vi "VFH.vi"(8 "Previous Calculated Sector":i16=90, 9 "Compass Bearing (degrees)":dbl, 10 "Target Bearing (degrees)":dbl, 11 "RAW SICK Data":T1) -> (3 "Calculated sector":i16)   [LabVIEW 2009]
uses:
  TypeDefs/Sensor TypeDefs/SICK Array.ctl
  Functional Global Variables/Actions for FG's.ctl
panel:
  in  "Roll offset":dbl
  in  "Pitch offset":dbl
  in  "Cost scaling factor":dbl=90.0
  in  "Heading scaling factor":dbl=5.0
  out "Number of Obstructed Sectors 3":i32
  out "Number of Obstructed Sectors 2":i32
  out "Number of Obstructed Sectors":i32
  out "Expansion Array 3":u16[](array[numeric])
  out "Expansion Array 2":u16[](array[numeric])
  out "Expansion Array":u16[](graph)
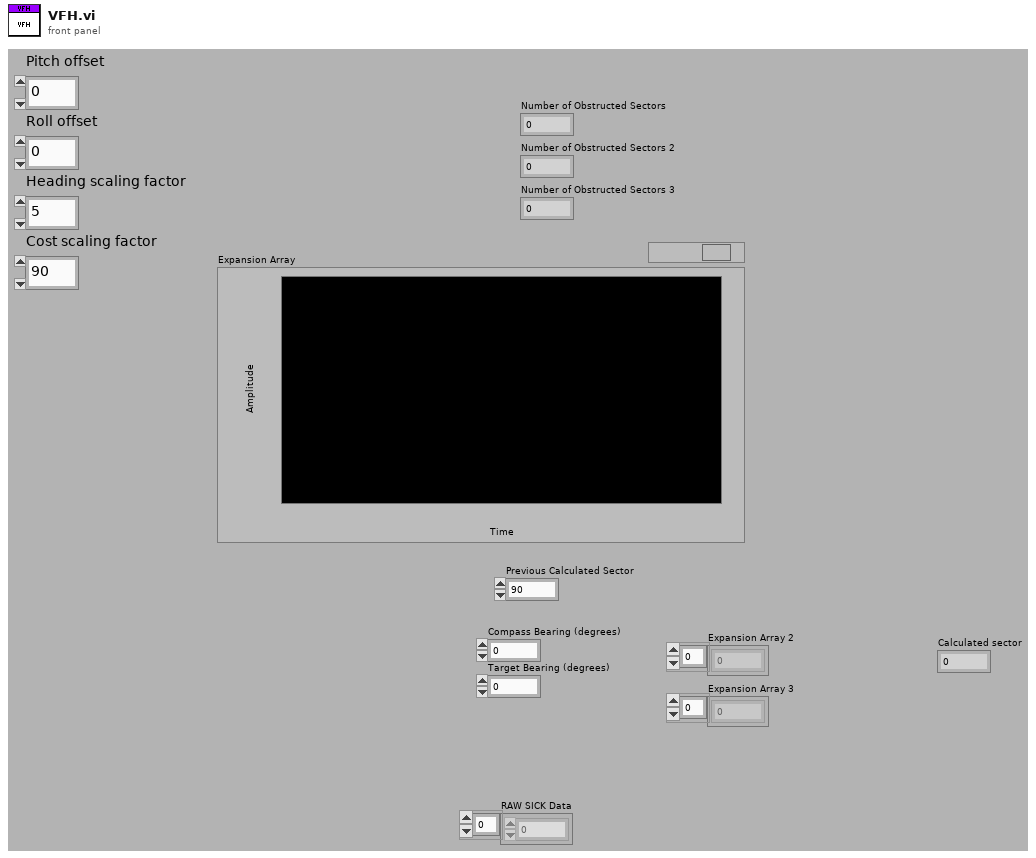
[diagram p1: front panel]
types:
  T1 = typedef "SICK Array.ctl" = u16[]
  T2 = typedef "Actions for FG's.ctl" = enum16{"Read", "Write"}
  T3 = typedef "VFH Parameters.ctl" = cluster{"Robot Radius":u16, "Near Threshold":u16, "Mid Threshold":u16, "Far Threshold":u16, "Weights":T4}
  T4 = typedef "VFH Weights.ctl" = cluster{"TS-S weight":dbl, "CS-S weight":dbl, "PCS-S weight":dbl, "Near weight":dbl, "Mid weight":dbl, "Far weight":dbl}
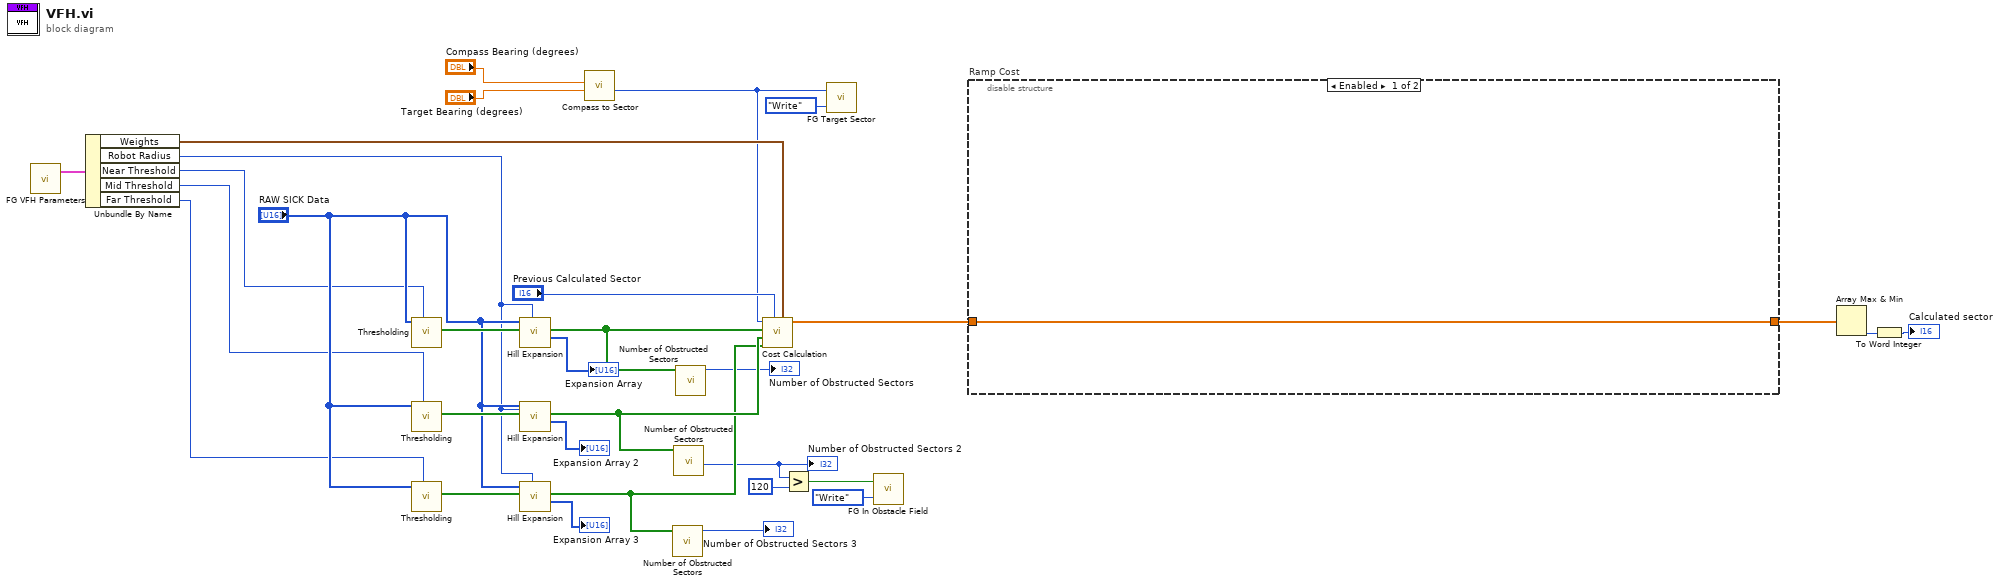
[diagram p0: block diagram]
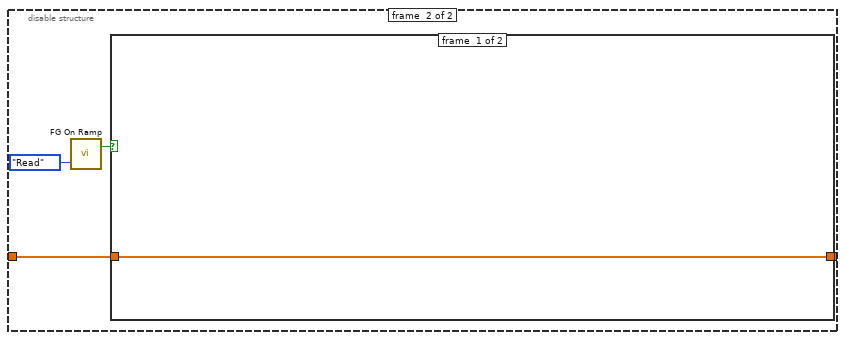
[diagram p2: hidden frame]
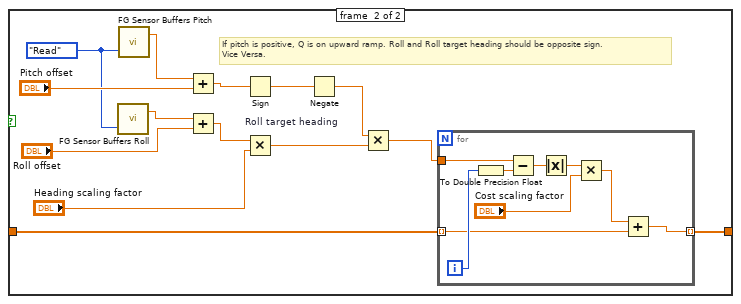
[diagram p3: hidden frame]
diagram:
  n1 = call "FG VFH Parameters.vi"() -> ("VFH Parameters out"=w23:T3)  [unwired: 3 in]
  n2 = Unbundle By Name(w23) -> ("Weights"=w18:T4, "Robot Radius"=w22:u16, "Near Threshold"=w21:u16, "Mid Threshold"=w20:u16, "Far Threshold"=w19:u16)
  n3 = call "Thresholding.vi"("Threshold"=w21, "RAW SICK Data"="RAW SICK Data") -> ("Boolean array"=w31:bool[])  [unwired: 1 in, 8 out]
  n4 = call "Thresholding.vi"("Threshold"=w20, "RAW SICK Data"="RAW SICK Data") -> ("Boolean array"=w29:bool[])  [unwired: 1 in, 8 out]
  n5 = call "Thresholding.vi"("Threshold"=w19, "RAW SICK Data"="RAW SICK Data") -> ("Boolean array"=w30:bool[])  [unwired: 1 in, 8 out]
  n6 = call "Hill Expansion.vi"("Robot Radius"=w22, "Boolean array"=w31, "RAW SICK Data"="RAW SICK Data") -> ("Expansion Array"=→"Expansion Array":u16[], "Expanded Boolean Array"=w11:bool[])  [unwired: 1 in, 6 out]
  n7 = call "Hill Expansion.vi"("Robot Radius"=w22, "Boolean array"=w29, "RAW SICK Data"="RAW SICK Data") -> ("Expansion Array"=→"Expansion Array 2":u16[], "Expanded Boolean Array"=w10:bool[])  [unwired: 1 in, 6 out]
  n8 = call "Hill Expansion.vi"("Robot Radius"=w22, "Boolean array"=w30, "RAW SICK Data"="RAW SICK Data") -> ("Expansion Array"=→"Expansion Array 3":u16[], "Expanded Boolean Array"=w9:bool[])  [unwired: 1 in, 6 out]
  n9 = call "Compass to Sector.vi"("Target Bearing (degrees)"="Target Bearing (degrees)", "Compass Bearing (degrees)"="Compass Bearing (degrees)") -> ("Target Heading (Sectors)"=w16:i16)  [unwired: 9 out]
  n10 = call "Number of Obstructed Sectors.vi"("Boolean Array"=w9) -> ("Number of Obstructed Sectors"=→"Number of Obstructed Sectors 3":i32)  [unwired: 10 in]
  n11 = call "Number of Obstructed Sectors.vi"("Boolean Array"=w10) -> ("Number of Obstructed Sectors"=w6:i32)  [unwired: 10 in]
  "Number of Obstructed Sectors 2" <- w6
  n12 = call "Number of Obstructed Sectors.vi"("Boolean Array"=w11) -> ("Number of Obstructed Sectors"=→"Number of Obstructed Sectors":i32)  [unwired: 10 in]
  n13 = call "Cost Calculation.vi"("Weights"=w18, "Previous Calculated Sector"="Previous Calculated Sector", "Far Boolean Array"=w9, "Mid Boolean Array"=w10, "Near Boolean Array"=w11, "Target Sector"=w16) -> ("Cost Array"=w2:dbl[])  [unwired: 5 in]
  n14 = Greater?(x=w6, y=120) -> (0:w4:bool)
  n15 = call "FG Target Sector.vi"("FG Action (Read)"=Actions_for_FG's."Write", "Target sector in"=w16) -> ()  [unwired: 1 in, 1 out]
  n16 = call "FG In Obstacle Field.vi"("FG Action (Read)"=Actions_for_FG's."Write", "In Obs. Field? in"=w4) -> ()  [unwired: 1 in, 1 out]
  n17 = disable-structure "Ramp Cost" shown="Enabled" {
    disable-tunnel: w2 -> [w32 w34]
    disable-tunnel: [w32 w33] -> w1
    frame #0 {
    }
    frame #1 {
      n18 = call "FG On Ramp.vi"("FG Action"=Actions_for_FG's."Read") -> ("On Ramp out"=w35:bool)  [unwired: 2 in]
      n19 = case shown="True" w35 {
        tunnel: w34 -> [w37 w50]
        tunnel: [w37 w49] -> w33
        frame #0 {
        }
        frame #1 {
          w42 = Actions_for_FG's."Read" ("FG Action (Read)")
          # "If pitch is positive, Q is on upward ramp. Roll and Roll target heading should be opposite sign.\nVice Versa."
          n20 = call "FG Sensor Buffers Roll.vi"("FG Action (Read)"=w42) -> ("Roll Buffer out"=w41:dbl)  [unwired: 2 in]
          n21 = call "FG Sensor Buffers Pitch.vi"("FG Action (Read)"=w42) -> ("Pitch Buffer out"=w44:dbl)  [unwired: 2 in]
          n22 = Add(x=w44, y="Pitch offset") -> (x+y=w39:dbl)
          n23 = Add(x=w41, y="Roll offset") -> (x+y=w38:dbl)
          n24 = Sign(1:w39) -> (0:w46:dbl)
          n25 = Multiply "Roll target heading"(x=w38, y="Heading scaling factor") -> (x*y=w48:dbl)
          n26 = Negate(x=w46) -> (-x=w47:dbl)
          n27 = Multiply(x=w47, y=w48) -> (x*y=w45:dbl)
          n28 = for {
            tunnel: w50 -> [w53] mode=indexing
            tunnel: w45 -> [w56]
            tunnel: [w52] -> w49 mode=indexing
            i -> [w59]
            n29 = To Double Precision Float(number=w59) -> (double precision float=w55:dbl)
            n30 = Subtract(x=w56, y=w55) -> (x-y=w60:dbl)
            n31 = Absolute Value(x=w60) -> (abs(x)=w58:dbl)
            n32 = Multiply(x=w58, y="Cost scaling factor") -> (x*y=w54:dbl)
            n33 = Add(x=w54, y=w53) -> (x+y=w52:dbl)
          }
        }
      }
    }
  }
  n34 = Array Max & Min(array=w1) -> (min index (indices)=w26:i32)  [unwired: 3 out]
  n35 = To Word Integer(number=w26) -> (16bit integer=→"Calculated sector":i16)
